vi "DAQ.TimedLoop.vi"(8 "error in (no error)":errorcluster, 11 "Instrument.DAQ in":refnum<class "Instrument.DAQ.lvclass">) -> (0 "error out":errorcluster, 3 "Instrument.DAQ out":refnum<class "Instrument.DAQ.lvclass">)   [LabVIEW 2019, in "Instrument.Lockin.lvlib" / "Instrument.DAQ.lvclass"]
uses:
  Instrument.DAQ.lvclass
  Typedefs/Set State-enum.ctl
  <vilib>/JKI/JKI SMO/SMO/SMO.lvclass
  C:/Program Files/National Instruments/LabVIEW 2019/vi.lib/JKI/JKI SMO/SMO/SMO.lvclass
panel:
  # "!!!!!!!!!!!!!!!!!!!!!!!!!!!!!!!!!!!!!!!!!!!!!!!!!!!!!!!!!!!!!!!!!!!!!!!!\nTHIS IS AN EXPERIMENTAL BLOCKING CALL TO:\nGenerate\nRead/Write\nDSP\nIt should listen to events that change AO or REF Channels.\nInside there is a timed loop that will not stop unless it receives events for Set State = stop; SMO Stop; or SMO error\n!!!!!!!!!!!!!!!!!!!!!!!!!!!!!!!!!!!!!!!!!!!!!!!!!!!!!!!!!!!!!!!!!!!!!"
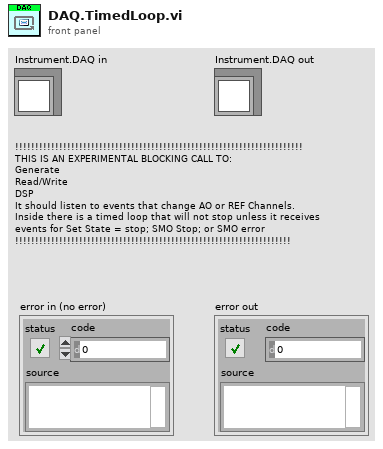
[diagram p1: front panel]
types:
  T1 = typedef "SMO.lvclass/Protected Events.ctl" = cluster{"StopProcesses":refnum<user-event>, "AbortProcesses":refnum<user-event>, "Config Changed":refnum<user-event>, "Dependency":refnum<user-event>}
  T2 = typedef "Instrument.Lockin.lvlib/Instrument.DAQ.lvclass/PrivateEvents--Cluster.ctl" = cluster{"setAOconfig":refnum<user-event>, "setAIconfig":refnum<user-event>, "setAO":refnum<user-event>, "setREF":refnum<user-event>, "setSampling":refnum<user-event>, "setState":refnum<user-event>, "setInputGain":refnum<user-event>, "setOutputGain":refnum<user-event>, "setSweep":refnum<user-event>, "measureOffset":refnum<user-event>, "zeroOffset":refnum<user-event>, "setPreFilter":refnum<user-event>, "autoConfigureDAQ":refnum<user-event>, "setCalibration":refnum<user-event>, "setAI":refnum<user-event>, "zeroPhase":refnum<user-event>, "setAmplitudeLimit":refnum<user-event>, "setLinkFrequencies":refnum<user-event>, "showUI":refnum<user-event>, "setInputOffset":refnum<user-event>, "setDCLimit":refnum<user-event>}
  T3 = typedef "Instrument.Lockin.lvlib/Instrument.DAQ.lvclass/Queue and Notifier.ctl" = cluster{"Message":refnum<queue>, "Instrument":refnum<queue>, "Stop":refnum<notifier>}
  T4 = typedef "Instrument.Lockin.lvlib/Instrument.DAQ.lvclass/Set State-enum.ctl" = enum16{"start", "stop", "reset", "start sweep", "stop sweep"}
  T5 = typedef "Instrument.Lockin.lvlib/Instrument.DAQ.lvclass/Results--Cluster.ctl" = cluster{"Time Stamp":timestamp, "Results (Dictionary)":cluster{"key":string, "value":dbl}[]}
  T6 = typedef "Instrument.Lockin.lvlib/Instrument.DAQ.lvclass/PublicEvents--DAQ.getWaveforms.ctl" = cluster{"AO_wfm":waveform(dbl)[], "AI_wfm":waveform(dbl)[], "Ref_X_wfm":waveform(dbl)[], "Ref_Y_wfm":waveform(dbl)[], "X_wfm":waveform(dbl)[], "Y_wfm":waveform(dbl)[]}
  T7 = typedef "Instrument.Lockin.lvlib/Instrument.DAQ.lvclass/AO.Channel--Cluster--Array.ctl" = T8[]
  T8 = typedef "Instrument.Lockin.lvlib/Instrument.DAQ.lvclass/AO.Channel--Cluster.ctl" = cluster{"Enable?":bool, "Channel":i32, "Amplitude":dbl, "Offset":dbl, "Frequency":dbl, "Phase":dbl, "Function":T9, "Sweeping?":bool, "Limit AC":bool, "Limit DC?":bool}
  T9 = typedef "Instrument.Lockin.lvlib/Instrument.DAQ.lvclass/AO.Channel.Function--Enum.ctl" = enum16{"Sine", "Triangle", "Square"}
  T10 = typedef "Instrument.Lockin.lvlib/Instrument.DAQ.lvclass/REF.Channel--Cluster--Array.ctl" = T11[]
  T11 = typedef "Instrument.Lockin.lvlib/Instrument.DAQ.lvclass/REF.Channel--Cluster.ctl" = cluster{"Enable?":bool, "Channel":i32, "Frequency":dbl, "Phase":dbl, "TC":dbl, "Roll-Off":i32}
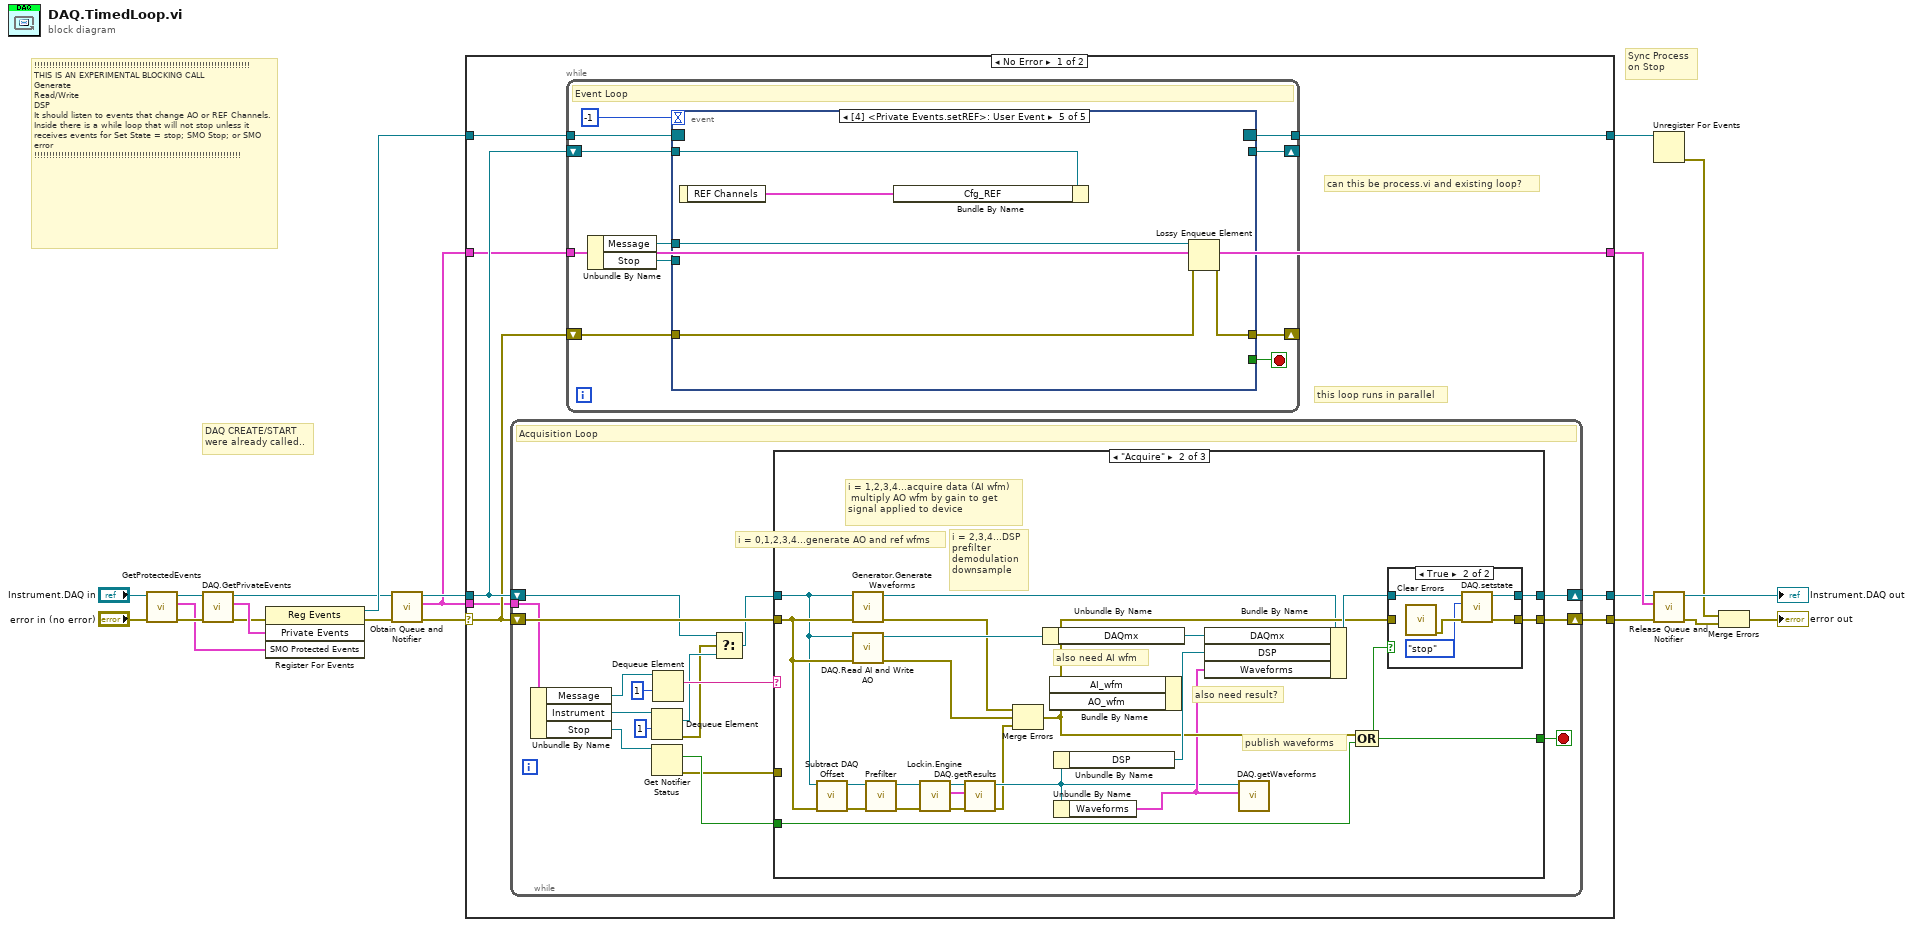
[diagram p0: block diagram]
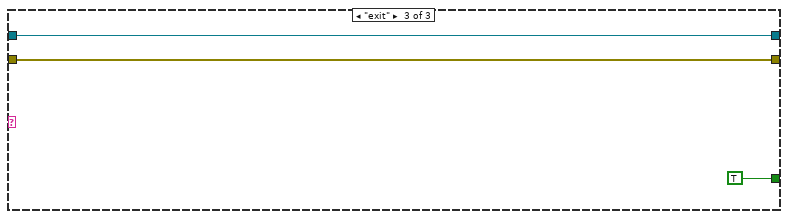
[diagram p4: hidden frame]
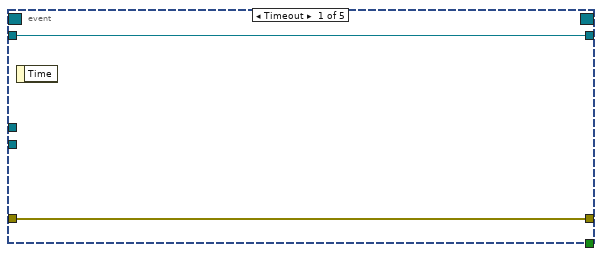
[diagram p5: hidden frame]
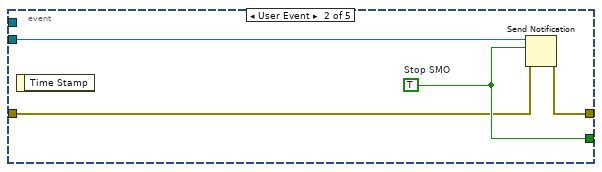
[diagram p6: hidden frame]
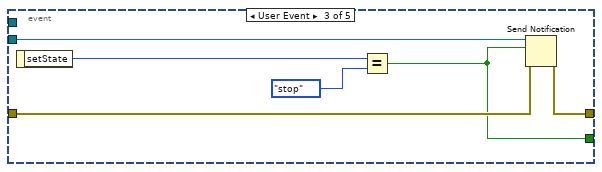
[diagram p7: hidden frame]
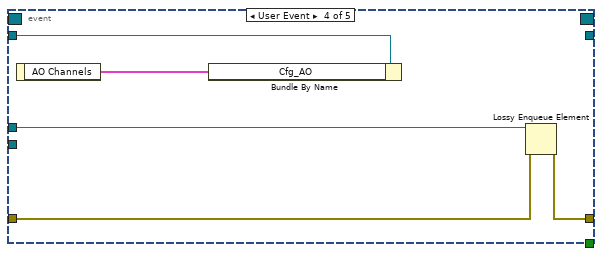
[diagram p8: hidden frame]
diagram:
  # "Sync Process\non Stop"
  # "DAQ CREATE/START\nwere already called.."
  # "!!!!!!!!!!!!!!!!!!!!!!!!!!!!!!!!!!!!!!!!!!!!!!!!!!!!!!!!!!!!!!!!!!!!!!!!\nTHIS IS AN EXPERIMENTAL BLOCKING CALL\nGenerate\nRead/Write\nDSP\nIt should listen to events that change AO or REF Channels.\nInside there is a while loop that will not stop unless it receives events for Set State = stop; SMO Stop; or SMO error\n!!!!!!!!!!!!!!!!!!!!!!!!!!!!!!!!!!!!!!!!!!!!!!!!!!!!!!!!!!!!!!!!!!!!!"
  n1 = call <vilib>:"GetProtectedEvents.vi"("error in (no error)"="error in (no error)", "SMO"="Instrument.DAQ in") -> ("error out"=w17:errorcluster, "SMO Protected Events"=w16:T1, "SMO out"=w18:refnum<class "Instrument.DAQ.lvclass">)  [unwired: 7 in]
  n2 = call "DAQ.GetPrivateEvents.vi"("error in (no error)"=w17, "Instrument.DAQ"=w18) -> ("error out"=w14:errorcluster, "Private Events"=w15:T2, "Instrument.DAQ"=w11:refnum<class "Instrument.DAQ.lvclass">)  [unwired: 7 in]
  n3 = register-events(error in=w14, w15, w16) -> (reference out=w13:refnum<event-registration>, error out=w12:errorcluster)  [unwired: 1 in]
  n4 = call "Obtain Queue and Notifier.vi"("error in (no error)"=w12, "Instrument.DAQ in"=w11) -> ("error out"=w9:errorcluster, "Queue and Notifier"=w8:T3, "Instrument.DAQ"=w10:refnum<class "Instrument.DAQ.lvclass">)  [unwired: 7 in]
  n5 = case shown="No Error" w9 {
    selector: w9 -> [w25 w117]
    tunnel: w10 -> [w26 w118]
    tunnel: w13 -> [w29 w119]
    tunnel: [w22 w117] -> w6
    tunnel: [w28 w119] -> w19
    tunnel: [w27 w118] -> w5
    tunnel: w8 -> [w23 w116]
    tunnel: w8 -> [w24 _]
    tunnel: [w23 w116] -> w7
    frame No Error {
      # "this loop runs in parallel"
      # "can this be process.vi and existing loop?"
      n6 = while {
        shift-right: [w46] -> w27
        shift-left: w26 -> [w32]
        shift-right: [w45] -> w22
        shift-left: w25 -> [w43]
        tunnel: w24 -> [w34]
        stop <- w44 stop-if-true
        # "Acquisition Loop"
        n7 = Unbundle By Name(w34) -> ("Message"=w35:refnum<queue>, "Instrument"=w41:refnum<queue>, "Stop"=w42:refnum<notifier>)
        n8 = Dequeue Element(queue=w41, timeout in ms (-1)=1) -> (element=w33:refnum<class "Instrument.DAQ.lvclass">, error out=w30:errorcluster)  [unwired: 1 in, 2 out]
        n9 = Get Notifier Status(notifier=w42) -> (current notification=w39:bool, error out=w38:errorcluster)  [unwired: 1 in, 3 out]
        n10 = Dequeue Element(queue=w35, timeout in ms (-1)=1) -> (element=w36:string)  [unwired: 1 in, 3 out]
        n11 = Select(t=w32, s=w30, f=w33) -> (s? t:f=w31:refnum<class "Instrument.DAQ.lvclass">)
        n12 = case shown="\"Acquire\"" w36 {
          tunnel: [w47 w71 w80] -> w46
          tunnel: [w48 w70 w81] -> w45
          tunnel: w31 -> [w47 w49 w80]
          tunnel: [_ w62 TRUE] -> w44
          tunnel: w43 -> [w48 w51 w81]
          tunnel: w39 -> [_ w52 _]
          tunnel: w38 -> [_ _ _]
          frame "idle" {
          }
          frame "Acquire" {
            # "i = 2,3,4...DSP\nprefilter\ndemodulation\ndownsample"
            # "i = 1,2,3,4...acquire data (AI wfm)\n multiply AO wfm by gain to get\nsignal applied to device"
            # "i = 0,1,2,3,4...generate AO and ref wfms"
            # "publish waveforms"
            # "also need result?"
            # "also need AI wfm"
            n13 = call "Subtract DAQ Offset.vi"("error in (no error)"=w51, "Instrument.DAQ"=w49) -> ("error out"=w53:errorcluster, "Instrument.DAQ out"=w60:refnum<class "Instrument.DAQ.lvclass">)  [unwired: 8 in]
            n14 = call "Generator.Generate Waveforms.vi"("error in (no error)"=w51, "Instrument.DAQ"=w49) -> ("error out"=w56:errorcluster, "Instrument.DAQ"=w55:refnum<class "Instrument.DAQ.lvclass">)  [unwired: 8 in]
            n15 = call "DAQ.Read AI and Write AO.vi"("error in (no error)"=w51, "Instrument.DAQ in"=w49) -> ("error out"=w63:errorcluster, "Instrument.DAQ out"=w67:refnum<class "Instrument.DAQ.lvclass">)  [unwired: 8 in]
            n16 = call "Prefilter.vi"("error in (no error)"=w53, "Instrument.DAQ in"=w60) -> ("error out"=w54:errorcluster, "Instrument.DAQ out"=w59:refnum<class "Instrument.DAQ.lvclass">)  [unwired: 8 in]
            n17 = call "Lockin.Engine.vi"("error in (no error)"=w54, "Instrument.DAQ"=w59) -> ("error out"=w69:errorcluster, "<Results> (X,Y,R,Theta,Mean)"=w72:T5, "Instrument.DAQ out"=w68:refnum<class "Instrument.DAQ.lvclass">)  [unwired: 7 in]
            n18 = call "DAQ.getResults.vi"("error in (no error)"=w69, "Results"=w72, "Instrument.DAQ"=w68) -> ("error out"=w50:errorcluster, "Instrument.DAQ out"=w57:refnum<class "Instrument.DAQ.lvclass">)  [unwired: 7 in]
            n19 = Merge Errors(w56, w63, w50) -> (w61:errorcluster)
            n20 = Unbundle By Name(w67) -> ("DAQmx"=w65:refnum<class "DAQmx.lvclass">)
            n21 = Bundle By Name() -> ()  [unwired: 3 in, 1 out]
            n22 = Unbundle By Name(w57) -> ("DSP"=w64:refnum<class "DSP.lvclass">)
            n23 = Unbundle By Name(w57) -> ("Waveforms"=w58:T6)
            n24 = Bundle By Name(cluster=w55, "DAQmx"=w65, "DSP"=w64, "Waveforms"=w58) -> (w66:refnum<class "Instrument.DAQ.lvclass">)
            n25 = call "DAQ.getWaveforms.vi"("Waveforms"=w58, "Instrument.DAQ"=w57) -> ()  [unwired: 8 in, 2 out]
            n26 = Compound Arithmetic op=OR(w61, w52) -> (w62:bool)
            n27 = case shown="True" w62 {
              tunnel: w66 -> [w74 w79]
              tunnel: [w74 w78] -> w71
              tunnel: [w73 w77] -> w70
              tunnel: w61 -> [w73 _]
              frame False {
              }
              frame True {
                n28 = call <vilib>:"Clear Errors.vi"() -> ("error out"=w76:errorcluster)  [unwired: 6 in, 1 out]
                n29 = call "DAQ.setstate.vi"("error in (no error)"=w76, "setState"=Set_State-enum."stop", "Instrument.DAQ"=w79) -> ("error out"=w77:errorcluster, "Instrument.DAQ out"=w78:refnum<class "Instrument.DAQ.lvclass">)  [unwired: 7 in]
              }
            }
          }
          frame "exit" {
          }
        }
      }
      n30 = while {
        tunnel: w29 -> [w93]
        tunnel: [w92] -> w28
        shift-right: [w86] -> _
        shift-left: w26 -> [w90]
        shift-right: [w88] -> _
        shift-left: w25 -> [w89]
        tunnel: w23 -> [w83]
        stop <- w91 stop-if-true
        # "Event Loop"
        n31 = Unbundle By Name(w83) -> ("Message"=w85:refnum<queue>, "Stop"=w84:refnum<notifier>)
        n32 = event shown="[4] <Private Events.setREF>: User Event" {
          selector: w93 -> [_ _ _ _ _]
          dyn-events: [_ _ _ _ _] -> w92
          timeout: -1 -> [_ _ _ _ _]
          tunnel: [_ w99 w100 _ _] -> w91
          tunnel: [w94 w97 w101 w110 w115] -> w88
          tunnel: w90 -> [w95 _ _ w107 w114]
          tunnel: w89 -> [w94 w98 w102 w108 w112]
          tunnel: [w95 _ _ _ _] -> w86
          tunnel: w85 -> [_ _ _ w106 w111]
          tunnel: w84 -> [_ w96 w103 _ _]
          event Timeout {
            n33 = event-data() -> ()  [unwired: 1 in, 1 out]
          }
          event User Event {
            w99 = TRUE  # Stop SMO
            n34 = event-data() -> ()  [unwired: 1 in, 1 out]
            n35 = Send Notification(notification=w99, notifier=w96, error in (no error)=w98) -> (error out=w97:errorcluster)  [unwired: 1 out]
          }
          event User Event {
            n36 = event-data() -> ("setState"=w105:T4)  [unwired: 1 in]
            n37 = Equal?(x=w105, y=Set_State-enum."stop") -> (x = y?=w100:bool)
            n38 = Send Notification(notification=w100, notifier=w103, error in (no error)=w102) -> (error out=w101:errorcluster)  [unwired: 1 out]
          }
          event User Event {
            n39 = event-data() -> ("AO Channels"=w109:T7)  [unwired: 1 in]
            n40 = Bundle By Name(cluster=w107, "Cfg_AO"=w109) -> ()  [unwired: 1 out]
            n41 = Lossy Enqueue Element(queue=w106, error in (no error)=w108) -> (error out=w110:errorcluster)  [unwired: 1 in, 3 out]
          }
          event User Event {
            n42 = event-data() -> ("REF Channels"=w113:T10)  [unwired: 1 in]
            n43 = Bundle By Name(cluster=w114, "Cfg_REF"=w113) -> ()  [unwired: 1 out]
            n44 = Lossy Enqueue Element(queue=w111, error in (no error)=w112) -> (error out=w115:errorcluster)  [unwired: 1 in, 3 out]
          }
        }
      }
    }
    frame Error {
    }
  }
  n45 = Unregister For Events(event registration refnum=w19) -> (error out=w2:errorcluster)  [unwired: 1 in]
  n46 = call "Release Queue and Notifier.vi"("error in (no error)"=w6, "Queue and Notifier"=w7, "Instrument.DAQ in"=w5) -> ("error out"=w1:errorcluster, "Instrument.DAQ out"=→"Instrument.DAQ out":refnum<class "Instrument.DAQ.lvclass">)  [unwired: 7 in]
  n47 = Merge Errors(w2, w1) -> (→"error out":errorcluster)
